vi "position traslation to name pos array.vi"(10 "Array":T2[](array[typedef])) -> (0 "name array":T1[](array[typedef]), 2 "pos array":cluster{"X":dbl, "Y":dbl}[](array[cluster]))   [LabVIEW 2019]
uses:
  ctl/position array.ctl
  ctl/position name.ctl
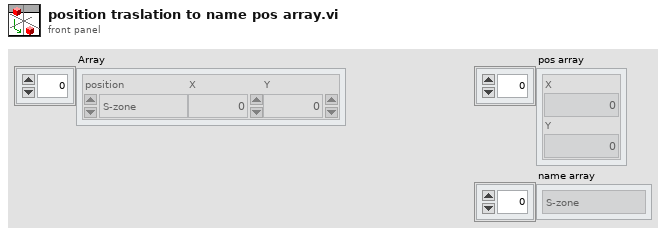
[diagram p1: front panel]
types:
  T1 = typedef "position name.ctl" = enum16{"S-zone", "out S", "vision board-vision", "out box", "box catch", "room center", "room right", "room left", "R2", "R4", "only rotate", "out recy", "recycle", "R3", "near board", "box poxition", "R1", "R5", "R1-d", "R5-d", "R3.4", "align center.1", "align center.5", "R2-d", "R2-r", "far center"}
  T2 = typedef "position array.ctl" = cluster{"position":T1, "X":dbl, "Y":dbl}
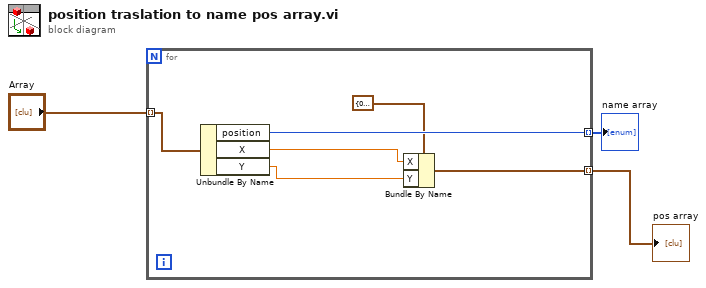
[diagram p0: block diagram]
diagram:
  n1 = for {
    tunnel: "Array" -> [w9] mode=indexing
    tunnel: [w8] -> w1 mode=indexing
    tunnel: [w4] -> w2 mode=indexing
    n2 = Unbundle By Name(w9) -> ("position"=w8:T1, "X"=w6:dbl, "Y"=w5:dbl)
    n3 = Bundle By Name(cluster=cluster{"X":dbl, "Y":dbl} {"X"=0.0, "Y"=0.0}, "X"=w6, "Y"=w5) -> (w4:cluster{"X":dbl, "Y":dbl})
  }
  "pos array" <- w2
  "name array" <- w1
